vi "[SubVI]Torque_Ramp.vi"(2 "Left Cadence Time":dbl, 3 "Right Cadence Time":dbl, 4 "Assistance Duration":dbl, 5 "Assistance Level (Nm)":dbl) -> (0 "Left Torque Profile":dbl[](array[numeric]), 1 "Right Torque Profile":dbl[](array[numeric]))   [LabVIEW 2018]
uses:
  <vilib>/Analysis/1siggen.llb/Ramp Pattern by Samples.vi
  <vilib>/Analysis/NI_AALBase.lvlib
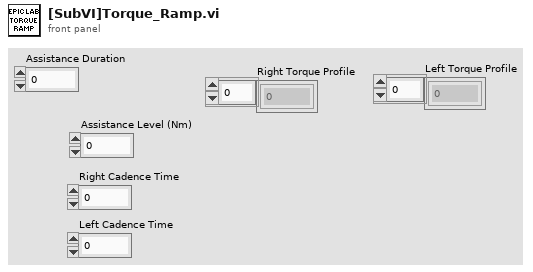
[diagram p1: front panel]
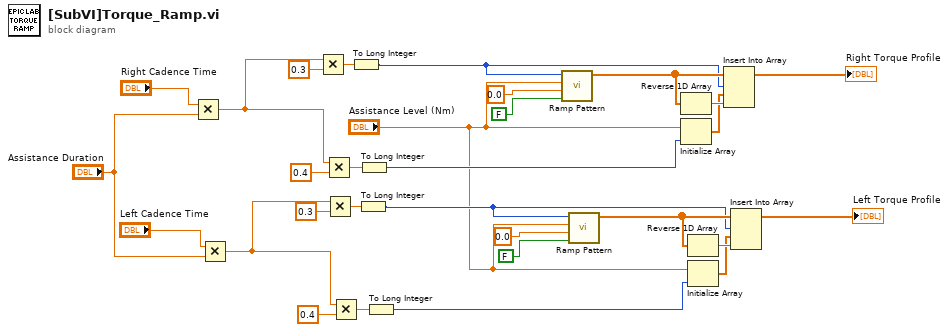
[diagram p0: block diagram]
diagram:
  n1 = Multiply(x="Right Cadence Time", y="Assistance Duration") -> (x*y=w18:dbl)
  n2 = Multiply(x="Left Cadence Time", y="Assistance Duration") -> (x*y=w4:dbl)
  n3 = Multiply(x=w18, y=0.3) -> (x*y=w22:dbl)
  n4 = Multiply(x=w18, y=0.4) -> (x*y=w20:dbl)
  n5 = Multiply(x=w4, y=0.3) -> (x*y=w8:dbl)
  n6 = Multiply(x=w4, y=0.4) -> (x*y=w6:dbl)
  n7 = To Long Integer(number=w22) -> (32bit integer=w21:i32)
  n8 = To Long Integer(number=w8) -> (32bit integer=w7:i32)
  n9 = To Long Integer(number=w20) -> (32bit integer=w19:i32)
  n10 = To Long Integer(number=w6) -> (32bit integer=w5:i32)
  n11 = call-poly <vilib>:"Ramp Pattern.vi"("exclude end?"=FALSE, "start"=0.0, "end"="Assistance Level (Nm)", "samples"=w21) -> ("Ramp Pattern"=w25:dbl[])  [unwired: 6 in, 1 out]
  n12 = call-poly <vilib>:"Ramp Pattern.vi"("exclude end?"=FALSE, "start"=0.0, "end"="Assistance Level (Nm)", "samples"=w7) -> ("Ramp Pattern"=w11:dbl[])  [unwired: 6 in, 1 out]
  n13 = Reverse 1D Array(array=w25) -> (reversed array=w28:dbl[])
  n14 = Initialize Array("Assistance Level (Nm)", w19) -> (w27:dbl[])
  n15 = Reverse 1D Array(array=w11) -> (reversed array=w14:dbl[])
  n16 = Initialize Array("Assistance Level (Nm)", w5) -> (w13:dbl[])
  n17 = Insert Into Array(array=w25, index=w21, new element #1=w27, new element #2=w28) -> (→"Right Torque Profile":dbl[])
  n18 = Insert Into Array(array=w11, index=w7, new element #1=w13, new element #2=w14) -> (→"Left Torque Profile":dbl[])
